vi "String Constant - Inside JKI SM Event Structure.vi"() -> ()   [LabVIEW 2020]
panel:
  in  "OK":bool
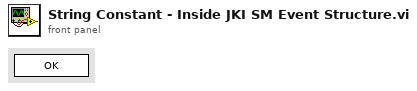
[diagram p1: front panel]
types:
  T1 = enum32{"invalid app kind", "Development System", "Run Time System", "Student Edition", "Embedded LabVIEW", "Evaluation", "Custom"}
  T2 = enum32{"Invalid", "Standard", "Closed", "Hidden", "Minimized", "Maximized"}
  T3 = cluster{"Core":cluster{"Current VI Reference":refnum<vi>, "Close Panel on Exit?":bool}, "Your Boolean data":bool}
  T4 = cluster{"Current VI Reference":refnum<vi>, "Close Panel on Exit?":bool}
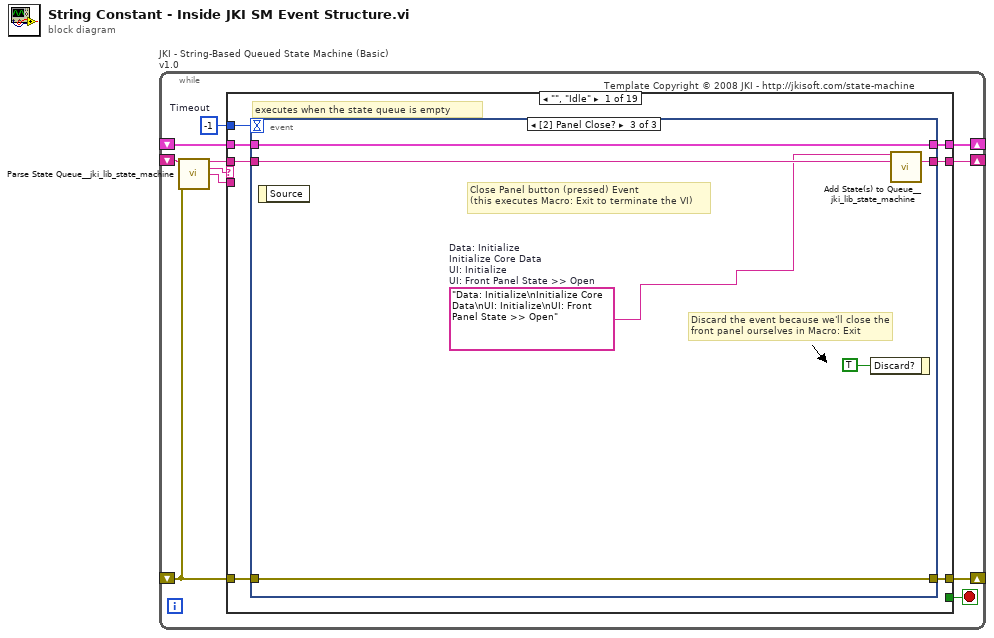
[diagram p0: block diagram]
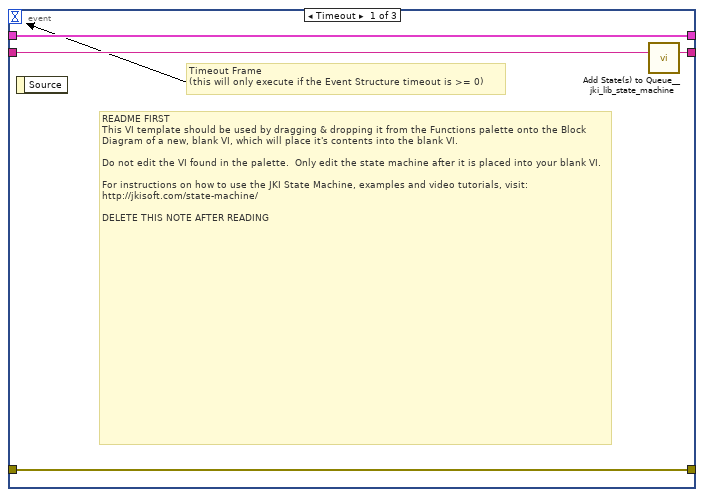
[diagram p2: hidden frame]
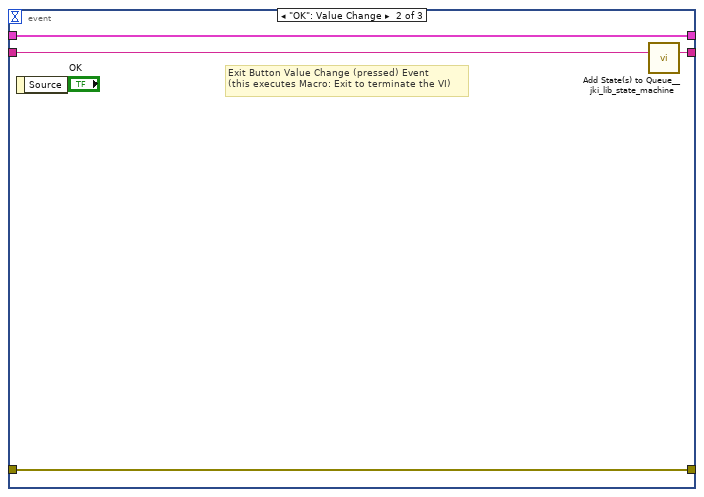
[diagram p3: hidden frame]
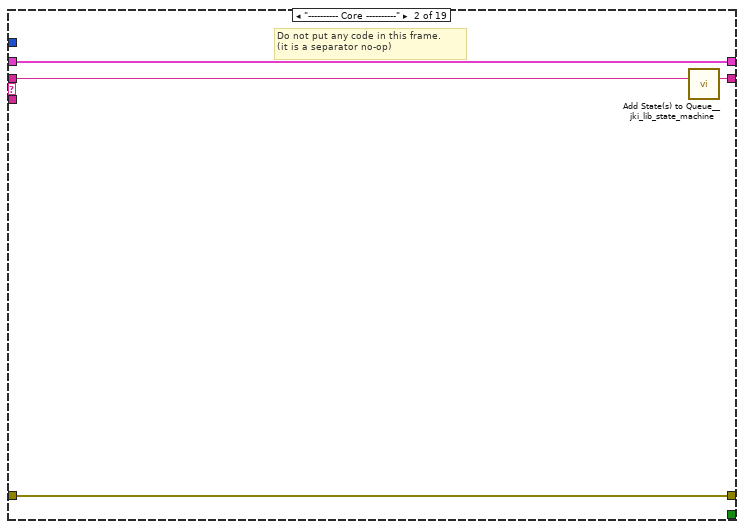
[diagram p4: hidden frame]
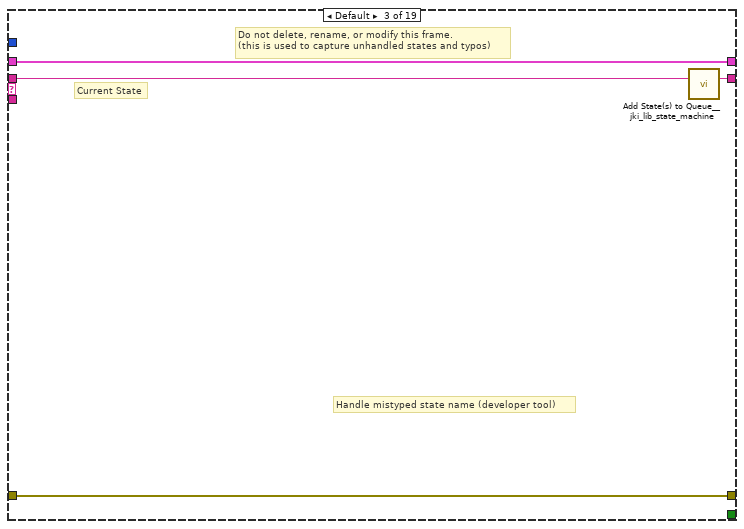
[diagram p5: hidden frame]
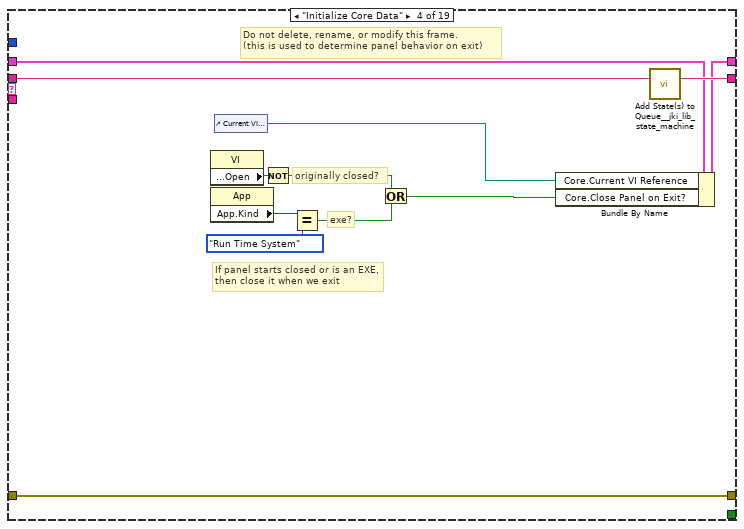
[diagram p6: hidden frame]
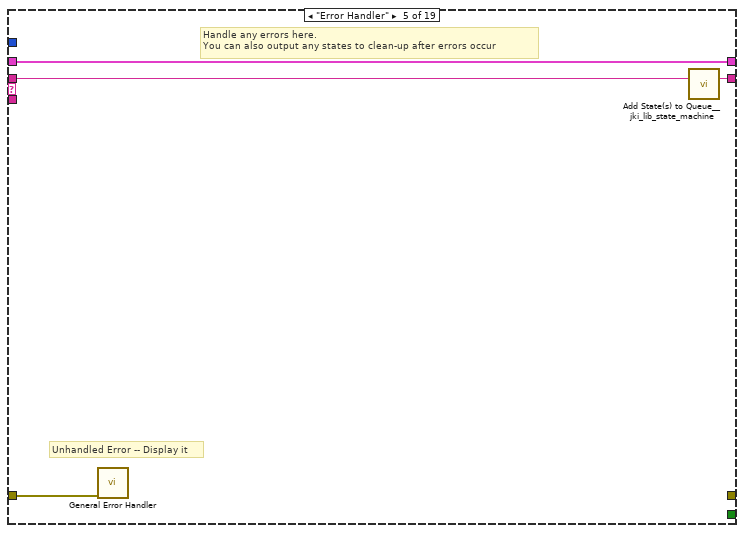
[diagram p7: hidden frame]
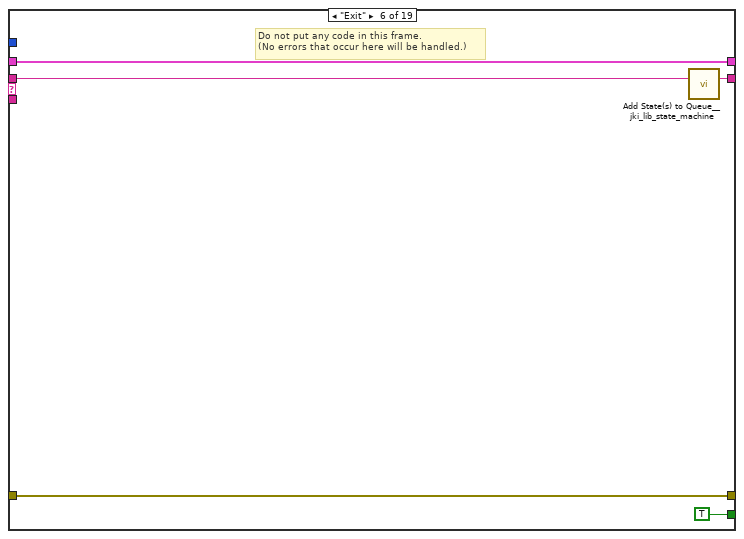
[diagram p8: hidden frame]
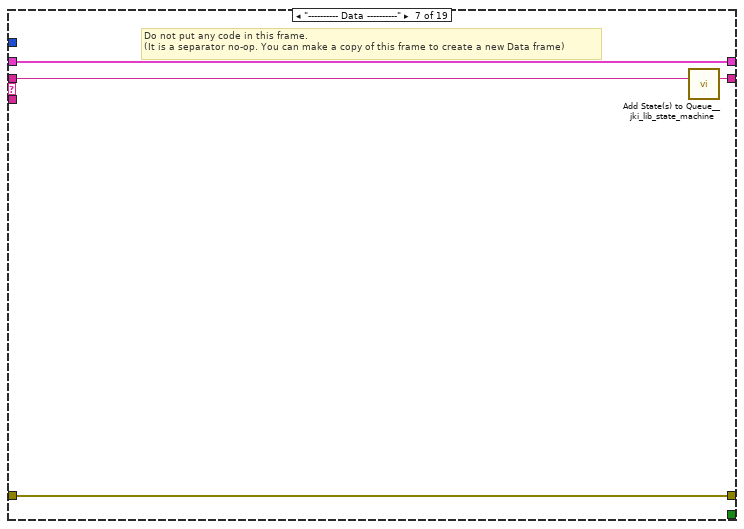
[diagram p9: hidden frame]
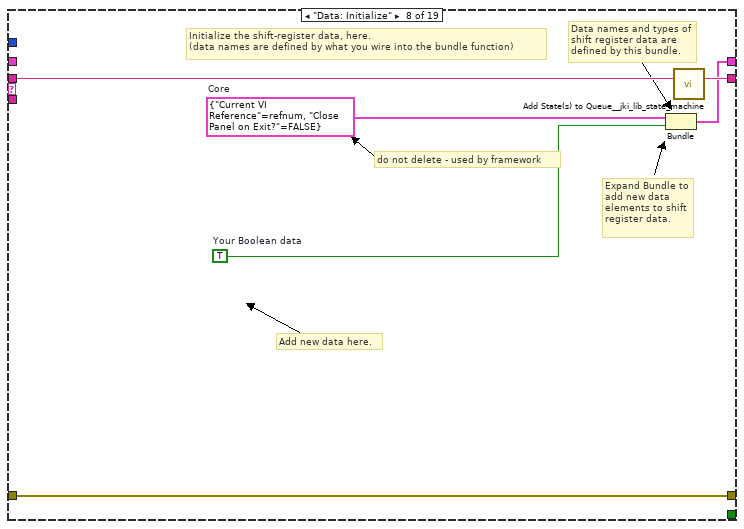
[diagram p10: hidden frame]
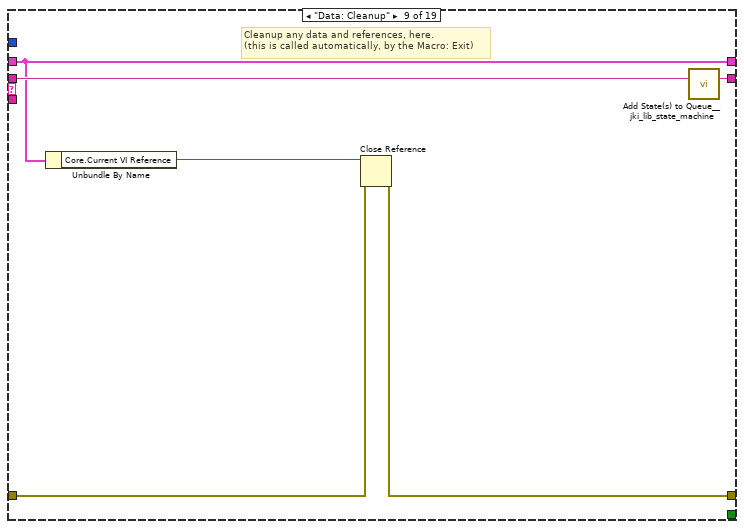
[diagram p11: hidden frame]
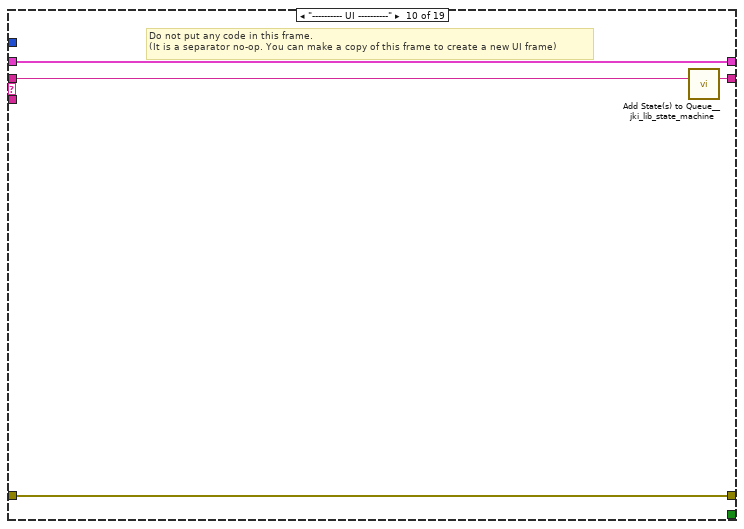
[diagram p12: hidden frame]
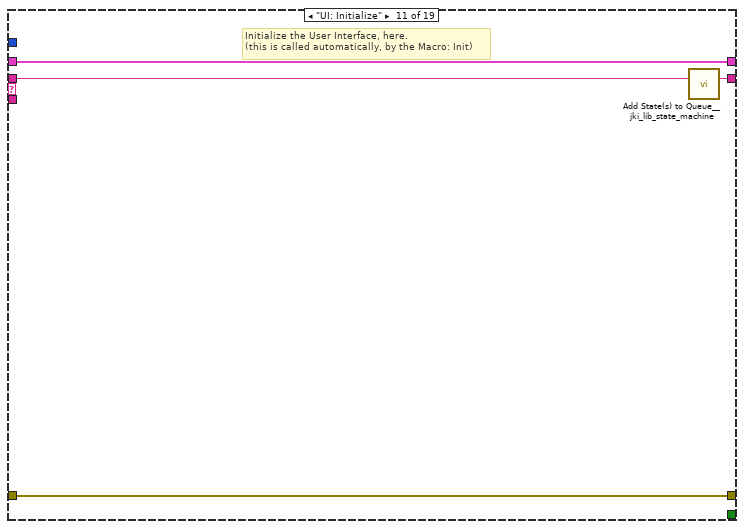
[diagram p13: hidden frame]
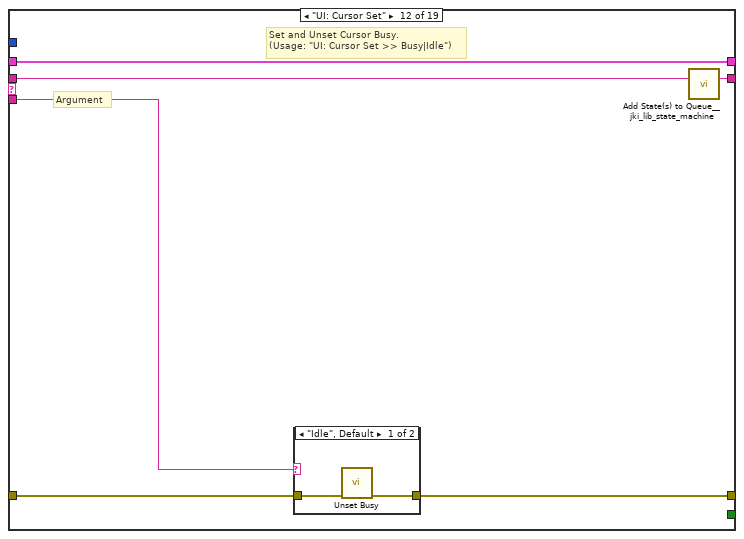
[diagram p14: hidden frame]
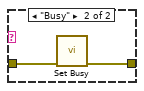
[diagram p15: hidden frame]
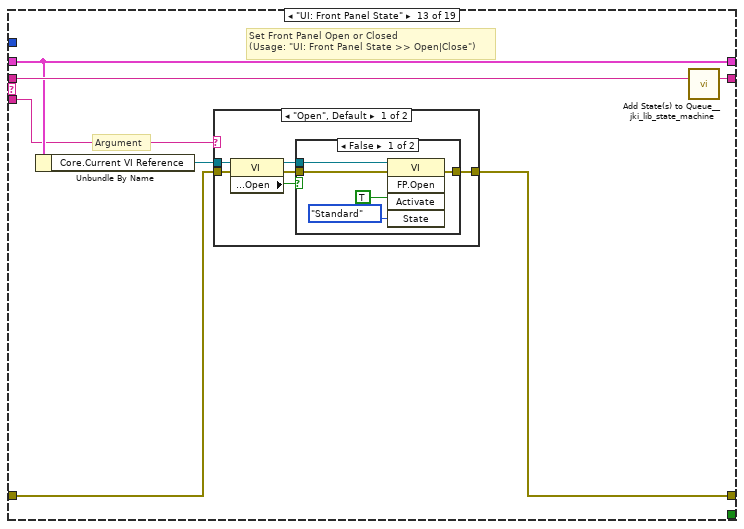
[diagram p16: hidden frame]
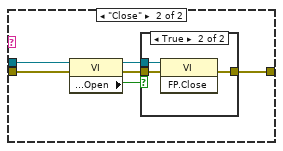
[diagram p18: hidden frame]
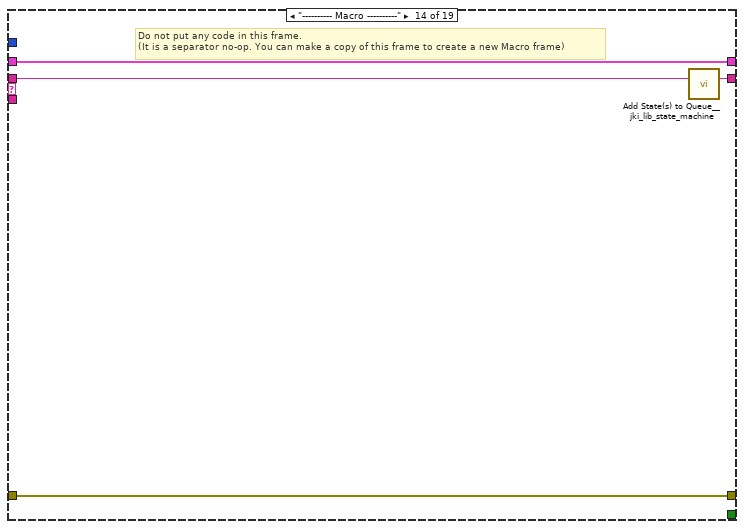
[diagram p20: hidden frame]
diagram:
  n1 = while "JKI - String-Based Queued State Machine (Basic) v1.0" {
    shift-right: [w4] -> _
    shift-left: _ -> [w3]
    shift-right: [w7] -> _
    shift-left: _ -> [w1]
    shift-right: [w6] -> _
    shift-left: _ -> [w8]
    stop <- w5 stop-if-true
    w2 = -1  # Timeout
    # "Template Copyright © 2008 JKI - http://jkisoft.com/state-machine"
    n2 = call <vilib>:"Parse State Queue__jki_lib_state_machine.vi"("State Queue"=w8, "Error In (no error)"=w1) -> ("Remaining States"=w10:string, "Current State"=w11:string, "Arguments"=w9:string)  [unwired: 11 in]
    n3 = case shown="\"\", \"Idle\"" w11 {
      tunnel: w10 -> [w18 w36 w39 w52 w56 w61 w65 w71 w77 w81 w85 w91 w102 w128 w132 w136 w140 w144 w148]
      tunnel: w9 -> [_ _ _ _ _ _ _ _ _ _ _ w86 w96 _ _ _ _ _ _]
      tunnel: w3 -> [w16 w33 w37 w43 w54 w59 w62 _ w72 w78 w83 w89 w98 w125 w129 w133 w137 w141 w145]
      tunnel: [w15 w34 w40 w49 _ w58 w63 w68 w73 w79 w82 w87 w99 w126 w130 w134 w138 w142 w146] -> w7
      tunnel: w1 -> [w14 w34 w40 w49 w53 w58 w63 w68 w74 w79 w82 w88 w100 w126 w130 w134 w138 w142 w146]
      tunnel: [w17 w35 w38 w51 w55 w60 w64 w70 w76 w80 w84 w90 w101 w127 w131 w135 w139 w143 w147] -> w6
      tunnel: [_ _ _ _ _ TRUE _ _ _ _ _ _ _ _ _ _ _ _ _] -> w5
      tunnel: [w13 w33 w37 w50 w54 w59 w62 w69 w72 w78 w83 w89 w98 w125 w129 w133 w137 w141 w145] -> w4
      tunnel: w2 -> [w12 _ _ _ _ _ _ _ _ _ _ _ _ _ _ _ _ _ _]
      frame "", "Idle" {
        # "executes when the state queue is empty"
        n4 = event shown="[2] Panel Close?" {
          selector: _ -> [_ _ _]
          dyn-events: _ -> [_ _ _]
          timeout: w12 -> [_ _ _]
          tunnel: w18 -> [w22 w26 w32]
          tunnel: [w21 w25 w31] -> w17
          tunnel: w16 -> [w19 w23 w29]
          tunnel: [w20 w24 w30] -> w15
          tunnel: w14 -> [w20 w24 w30]
          tunnel: [w19 w23 w29] -> w13
          event Timeout {
            # "README FIRST\nThis VI template should be used by dragging & dropping it from the Functions palette onto the Block Diagram of a new, blank VI, which will place it's contents into the blank VI.\n\nDo not edit the VI found in the palette.  Only edit the state machine after it is placed into your blank VI.\n\nFor instructions on how to use the JKI State Machine, examples and video tutorials, visit:\nhttp://jkisoft.com/state-machine/\n\nDELETE THIS NOTE AFTER READING"
            # "Timeout Frame\n(this will only execute if the Event Structure timeout is >= 0)"
            n5 = event-data() -> ()  [unwired: 1 in, 1 out]
            n6 = call <vilib>:"Add State(s) to Queue__jki_lib_state_machine.vi"("State(s) in (\"\")"=w22) -> ("States Out"=w21:string)  [unwired: 14 in]
          }
          event "OK": Value Change {
            # "Exit Button Value Change (pressed) Event\n(this executes Macro: Exit to terminate the VI)"
            n7 = event-data() -> ()  [unwired: 1 in, 1 out]
            n8 = call <vilib>:"Add State(s) to Queue__jki_lib_state_machine.vi"("State(s) in (\"\")"=w26) -> ("States Out"=w25:string)  [unwired: 14 in]
          }
          event Panel Close? {
            w27 = "Data: Initialize\nInitialize Core Data\nUI: Initialize\nUI: Front Panel State >> Open"  # Data: Initialize Initialize Core Data UI: Initialize UI: Front Panel State >> Open
            # "Discard the event because we'll close the front panel ourselves in Macro: Exit"
            # "Close Panel button (pressed) Event\n(this executes Macro: Exit to terminate the VI)"
            n9 = event-data() -> ()  [unwired: 1 in, 1 out]
            n10 = event-data("Discard?"=TRUE) -> ()  [unwired: 1 in, 1 out]
            n11 = call <vilib>:"Add State(s) to Queue__jki_lib_state_machine.vi"("State(s) in Front (\"\")"=w27, "State(s) in (\"\")"=w32) -> ("States Out"=w31:string)  [unwired: 13 in]
          }
        }
      }
      frame "---------- Core ----------" {
        # "Do not put any code in this frame.\n(it is a separator no-op)"
        n12 = call <vilib>:"Add State(s) to Queue__jki_lib_state_machine.vi"("State(s) in (\"\")"=w36) -> ("States Out"=w35:string)  [unwired: 14 in]
      }
      frame Default {
        # "Current State"
        # "Do not delete, rename, or modify this frame.\n(this is used to capture unhandled states and typos)"
        # "Handle mistyped state name (developer tool)"
        n13 = call <vilib>:"Add State(s) to Queue__jki_lib_state_machine.vi"("State(s) in (\"\")"=w39) -> ("States Out"=w38:string)  [unwired: 14 in]
      }
      frame "Initialize Core Data" {
        # "Do not delete, rename, or modify this frame.\n(this is used to determine panel behavior on exit)"
        # "originally closed?"
        # "exe?"
        # "If panel starts closed or is an EXE, then close it when we exit"
        n14 = property class="VI"() -> ("Front Panel.Open"=w48:bool)  [unwired: 2 in, 2 out]
        n15 = property class="App"() -> ("App.Kind"=w47:T1)  [unwired: 2 in, 2 out]
        n16 = control-ref of="Current VI Reference"() -> (w41:refnum<vi>)
        n17 = Not(x=w48) -> (.not. x?=w45:bool)
        n18 = Equal?(x=w47, y=T1."Run Time System" ("Application:Kind")) -> (x = y?=w44:bool)
        n19 = Or(x=w45, y=w44) -> (x .or. y?=w42:bool)
        n20 = Bundle By Name(cluster=w43, "Core.Current VI Reference"=w41, "Core.Close Panel on Exit?"=w42) -> (w50:T3)
        n21 = call <vilib>:"Add State(s) to Queue__jki_lib_state_machine.vi"("State(s) in (\"\")"=w52) -> ("States Out"=w51:string)  [unwired: 14 in]
      }
      frame "Error Handler" {
        # "Unhandled Error -- Display it"
        # "Handle any errors here.\nYou can also output any states to clean-up after errors occur"
        n22 = call <vilib>:"General Error Handler.vi"("error in (no error)"=w53) -> ()  [unwired: 10 in, 5 out]
        n23 = call <vilib>:"Add State(s) to Queue__jki_lib_state_machine.vi"("State(s) in (\"\")"=w56) -> ("States Out"=w55:string)  [unwired: 14 in]
      }
      frame "Exit" {
        # "Do not put any code in this frame.\n(No errors that occur here will be handled.)"
        n24 = call <vilib>:"Add State(s) to Queue__jki_lib_state_machine.vi"("State(s) in (\"\")"=w61) -> ("States Out"=w60:string)  [unwired: 14 in]
      }
      frame "---------- Data ----------" {
        # "Do not put any code in this frame.\n(It is a separator no-op. You can make a copy of this frame to create a new Data frame)"
        n25 = call <vilib>:"Add State(s) to Queue__jki_lib_state_machine.vi"("State(s) in (\"\")"=w65) -> ("States Out"=w64:string)  [unwired: 14 in]
      }
      frame "Data: Initialize" {
        w66 = T4 {"Current VI Reference"=refnum, "Close Panel on Exit?"=FALSE}  # Core
        w67 = TRUE  # Your Boolean data
        # "do not delete - used by framework"
        # "Expand Bundle to add new data elements to shift register data."
        # "Add new data here."
        # "Data names and types of shift register data are defined by this bundle."
        # "Initialize the shift-register data, here.\n(data names are defined by what you wire into the bundle function)"
        n26 = Bundle("Core"=w66, "Your Boolean data"=w67) -> (w69:T3)  [unwired: 1 in]
        n27 = call <vilib>:"Add State(s) to Queue__jki_lib_state_machine.vi"("State(s) in (\"\")"=w71) -> ("States Out"=w70:string)  [unwired: 14 in]
      }
      frame "Data: Cleanup" {
        # "Cleanup any data and references, here.\n(this is called automatically, by the Macro: Exit)"
        n28 = Unbundle By Name(w72) -> ("Core.Current VI Reference"=w75:refnum<vi>)
        n29 = Close Reference(reference=w75, error in (no error)=w74) -> (error out=w73:errorcluster)
        n30 = call <vilib>:"Add State(s) to Queue__jki_lib_state_machine.vi"("State(s) in (\"\")"=w77) -> ("States Out"=w76:string)  [unwired: 14 in]
      }
      frame "---------- UI ----------" {
        # "Do not put any code in this frame.\n(It is a separator no-op. You can make a copy of this frame to create a new UI frame)"
        n31 = call <vilib>:"Add State(s) to Queue__jki_lib_state_machine.vi"("State(s) in (\"\")"=w81) -> ("States Out"=w80:string)  [unwired: 14 in]
      }
      frame "UI: Initialize" {
        # "Initialize the User Interface, here.\n(this is called automatically, by the Macro: Init)"
        n32 = call <vilib>:"Add State(s) to Queue__jki_lib_state_machine.vi"("State(s) in (\"\")"=w85) -> ("States Out"=w84:string)  [unwired: 14 in]
      }
      frame "UI: Cursor Set" {
        # "Argument"
        # "Set and Unset Cursor Busy.\n(Usage: \"UI: Cursor Set >> Busy|Idle\")"
        n33 = case shown="\"Idle\", Default" w86 {
          tunnel: w88 -> [w93 w95]
          tunnel: [w92 w94] -> w87
          frame "Idle", Default {
            n34 = call <vilib>:"Unset Busy.vi"("error in (no error)"=w93) -> ("error out"=w92:errorcluster)  [unwired: 10 in]
          }
          frame "Busy" {
            n35 = call <vilib>:"Set Busy.vi"("error in (no error)"=w95) -> ("error out"=w94:errorcluster)  [unwired: 9 in, 1 out]
          }
        }
        n36 = call <vilib>:"Add State(s) to Queue__jki_lib_state_machine.vi"("State(s) in (\"\")"=w91) -> ("States Out"=w90:string)  [unwired: 14 in]
      }
      frame "UI: Front Panel State" {
        # "Argument"
        # "Set Front Panel Open or Closed\n(Usage: \"UI: Front Panel State >> Open|Close\")"
        n37 = Unbundle By Name(w98) -> ("Core.Current VI Reference"=w97:refnum<vi>)
        n38 = case shown="\"Open\", Default" w96 {
          tunnel: w100 -> [w106 w119]
          tunnel: [w108 w120] -> w99
          tunnel: w97 -> [w107 w117]
          frame "Open", Default {
            n39 = property class="VI"(reference=w107, error in=w106) -> (reference out=w104:refnum<vi>, error out=w105:errorcluster, "Front Panel.Open"=w103:bool)
            n40 = case shown="False" w103 {
              tunnel: [w111 w114] -> w108
              tunnel: w105 -> [w110 w114]
              tunnel: w104 -> [w109 _]
              frame False {
                n41 = invoke class="VI" method="FP.Open"(reference=w109, error in=w110, "Activate"=TRUE, "State"=T2."Standard") -> (error out=w111:errorcluster)  [unwired: 1 in, 4 out]
              }
              frame True {
              }
            }
          }
          frame "Close" {
            n42 = property class="VI"(reference=w117, error in=w119) -> (reference out=w116:refnum<vi>, error out=w118:errorcluster, "Front Panel.Open"=w115:bool)
            n43 = case shown="True" w115 {
              tunnel: [w121 w124] -> w120
              tunnel: w118 -> [w121 w123]
              tunnel: w116 -> [_ w122]
              frame False {
              }
              frame True {
                n44 = invoke class="VI" method="FP.Close"(reference=w122, error in=w123) -> (error out=w124:errorcluster)  [unwired: 1 in, 2 out]
              }
            }
          }
        }
        n45 = call <vilib>:"Add State(s) to Queue__jki_lib_state_machine.vi"("State(s) in (\"\")"=w102) -> ("States Out"=w101:string)  [unwired: 14 in]
      }
      frame "---------- Macro ----------" {
        # "Do not put any code in this frame.\n(It is a separator no-op. You can make a copy of this frame to create a new Macro frame)"
        n46 = call <vilib>:"Add State(s) to Queue__jki_lib_state_machine.vi"("State(s) in (\"\")"=w128) -> ("States Out"=w127:string)  [unwired: 14 in]
      }
      frame "Macro: Initialize" {
        # "Initialization Macro\n(This is called once, when the VI starts)"
        n47 = call <vilib>:"Add State(s) to Queue__jki_lib_state_machine.vi"("State(s) in (\"\")"=w132) -> ("States Out"=w131:string)  [unwired: 14 in]
      }
      frame "Macro: Exit" {
        # "Exit Macro\n(This is called once, when the VI exits)"
        n48 = Unbundle By Name(w133) -> ()  [unwired: 1 out]
        n49 = call <vilib>:"Add State(s) to Queue__jki_lib_state_machine.vi"("State(s) in (\"\")"=w136) -> ("States Out"=w135:string)  [unwired: 14 in]
      }
      frame "---------- New Category ----------" {
        # "Template Separator\n(You can make a copy of, or modify, this frame)"
        n50 = call <vilib>:"Add State(s) to Queue__jki_lib_state_machine.vi"("State(s) in (\"\")"=w140) -> ("States Out"=w139:string)  [unwired: 14 in]
      }
      frame "New Category: 1" {
        # "Your code here.\n(You can make a copy of, or modify, this frame)"
        n51 = call <vilib>:"Add State(s) to Queue__jki_lib_state_machine.vi"("State(s) in (\"\")"=w144) -> ("States Out"=w143:string)  [unwired: 14 in]
      }
      frame "New Category: 2" {
        # "Your code here.\n(You can make a copy of, or modify, this frame)"
        n52 = call <vilib>:"Add State(s) to Queue__jki_lib_state_machine.vi"("State(s) in (\"\")"=w148) -> ("States Out"=w147:string)  [unwired: 14 in]
      }
    }
  }
